vi "CreatePublicEvents.vi"(8 "error in (no error)":errorcluster, 11 "SMO":refnum<class "SMO.lvclass">) -> (0 "error out":errorcluster, 3 "SMO out":refnum<class "SMO.lvclass">)   [LabVIEW 2013, in "SMO.lvclass"]
uses:
  SMO.lvclass
  Typedefs/SMOState --Enum.ctl
  SMO.lvclass/SMO.ctl
panel:
  # "For instructions on how to use the JKI State Machine Objects, examples and video tutorials, visit:\nhttp://jki.net/state-machine-objects/\n\nJKI State Machine Objects™\nhttp://jki.net/state-machine-objects/\nCopyright (C) 2005-2015, JKI <info@jki.net>\nALL RIGHTS RESERVED"
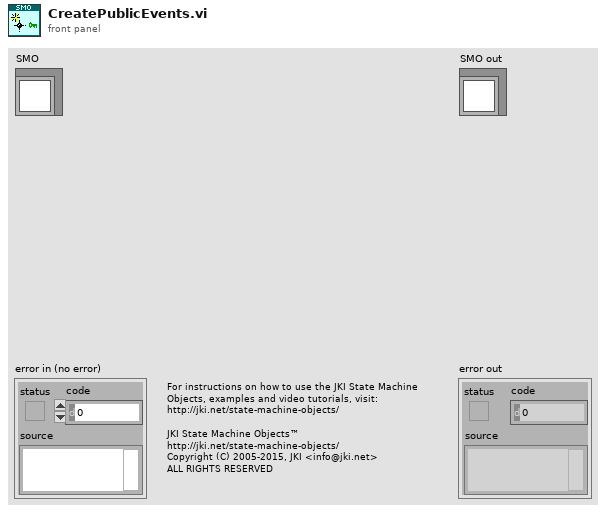
[diagram p1: front panel]
types:
  T1 = typedef "SMO.lvclass/SMOState --Enum.ctl" = enum16{"unknown", "Created", "Started", "Stopped"}
  T2 = cluster{"error":refnum<user-event>, "SMO State":refnum<user-event>}
  T3 = typedef "SMO.lvclass/PrivateData--Ref.ctl" = refnum<data-value>
  T4 = typedef "SMO.lvclass/PrivateData--Cluster.ctl" = cluster{"SMO Name":string, "Parent Call":T5, "Registered Processes":T6[], "Sync Notifier":refnum<notifier>, "Process Error Notifier":refnum<notifier>, "Protected Events":T7, "Public Events":T8, "SMO State":T1}
  T5 = typedef "SMO.lvclass/Parent Call--Enum.ctl" = enum16{"Allows parent to run", "Does not request parent to run"}
  T6 = typedef "SMO.lvclass/RegisteredProcessData--Cluster.ctl" = cluster{"Name":string, "Static VI Ref":refnum<vi>, "Running":bool, "NotifierRef":u32}
  T7 = typedef "SMO.lvclass/Protected Events.ctl" = cluster{"StopProcesses":refnum<user-event>, "AbortProcesses":refnum<user-event>}
  T8 = typedef "SMO.lvclass/Public Events.ctl" = cluster{"Error":refnum<user-event>, "State":refnum<user-event>}
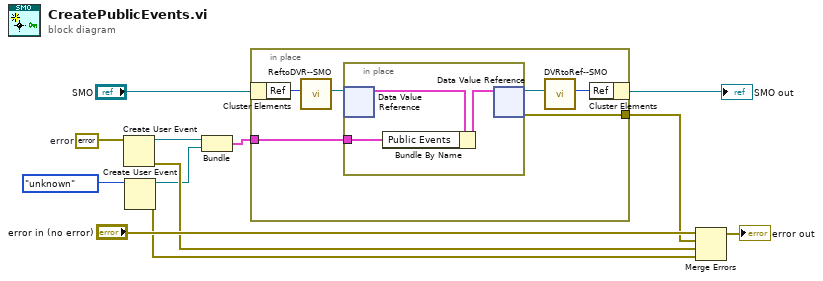
[diagram p0: block diagram]
diagram:
  w5 = errorcluster {"status"=FALSE, "code"=0, "source"=""}  # error
  n1 = Create User Event(user event datatype=w5) -> (user event=w6:refnum<user-event>, error out=w4:errorcluster)  [unwired: 1 in]
  n2 = Create User Event(user event datatype=SMOState_--Enum."unknown" ("SMO State")) -> (user event=w2:refnum<user-event>, error out=w1:errorcluster)  [unwired: 1 in]
  n3 = Bundle("error"=w6, "SMO State"=w2) -> (w7:T2)  [unwired: 1 in]
  n4 = in-place {
    in-place-border: w7 -> [w18]
    in-place-border: [w17] -> w8
    n5 = in-place-cluster #1("SMO") -> ("Ref"=w16:u32)
    n6 = call "ReftoDVR--SMO.vi"("Ref"=w16) -> ("Ref"=w15:T3)  [unwired: 10 in]
    n7 = in-place {
      in-place-border: w18 -> [w19]
      n8 = in-place-dvr #2(w15) -> (w21:T4)  [unwired: 1 out]
      n9 = Bundle By Name(cluster=w21, "Public Events"=w19) -> (w20:T4)
      n10 = in-place-dvr #2(w20) -> (w14:T3, w17:errorcluster)
    }
    n11 = call "DVRtoRef--SMO.vi"("Ref"=w14) -> ("Ref"=w13:u32)  [unwired: 10 in]
    n12 = in-place-cluster #1("Ref"=w13) -> (→"SMO out":refnum<class "SMO.lvclass">)
  }
  n13 = Merge Errors("error in (no error)", w8, w4, w1) -> (→"error out":errorcluster)
